vi "Copy_SourceItem.vi"(7 "referencedNonLVTypeMembers in":T1[](array[typedef]), 8 "error in (no error)":errorcluster, 10 "AB_Build.lvclass":refnum<class "AB_Build.lvclass">, 11 "AB_Source_ExportedVI in":refnum<class "AB_Source_ExportedVI.lvclass">) -> (0 "error out":errorcluster, 1 "newFileFlags":T2, 2 "newFileInfo":T3, 3 "AB_Source_ExportedVI out":refnum<class "AB_Source_ExportedVI.lvclass">, 5 "referencedNonLVTypeMembers out":T1[](array[typedef]))   [LabVIEW 2020, in "AB_Source_ExportedVI.lvclass"]
uses:
  <vilib>/AppBuilder/AB_Classes/Source/ExportedVI/AB_Source_ExportedVI.lvclass
  <vilib>/AppBuilder/AB_Classes/Build/AB_Build.lvclass
  <vilib>/AppBuilder/Engine/AB_Engine_New_File_Info.ctl
  <vilib>/AppBuilder/Engine/AB_Engine_New_File_Flags.ctl
  <vilib>/AppBuilder/AB_Source_Referenced_Libray_Files.ctl
  <vilib>/AppBuilder/AB_Classes/Source/VI/AB_Source_VI.lvclass
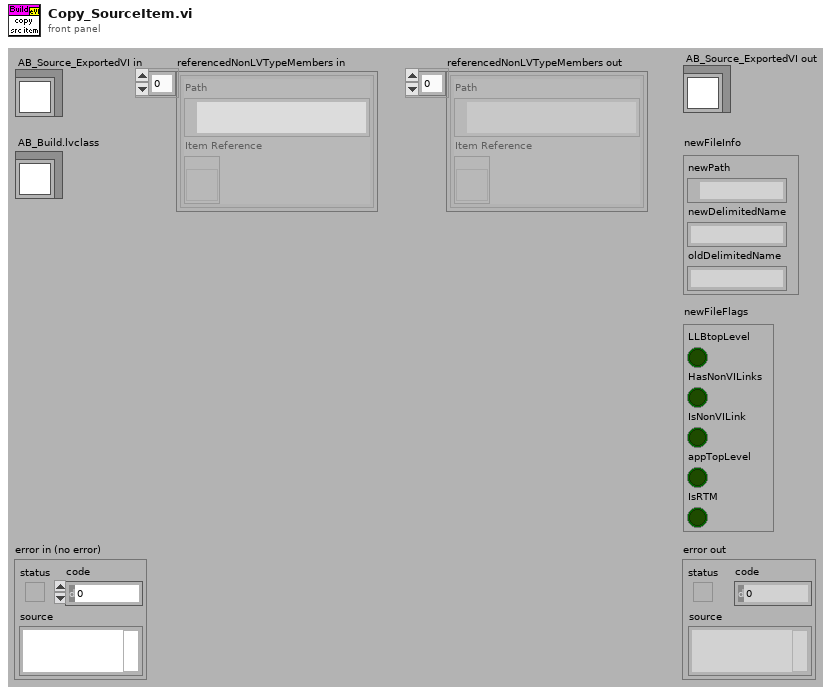
[diagram p1: front panel]
types:
  T1 = typedef "AB_Source_Referenced_Libray_Files.ctl" = cluster{"Path":path, "Item Reference":refnum<vi>}
  T2 = typedef "AB_Engine_New_File_Flags.ctl" = cluster{"LLBtopLevel":bool, "HasNonVILinks":bool, "IsNonVILink":bool, "appTopLevel":bool, "IsRTM":bool}
  T3 = typedef "AB_Engine_New_File_Info.ctl" = cluster{"newPath":path, "newDelimitedName":string, "oldDelimitedName":string}
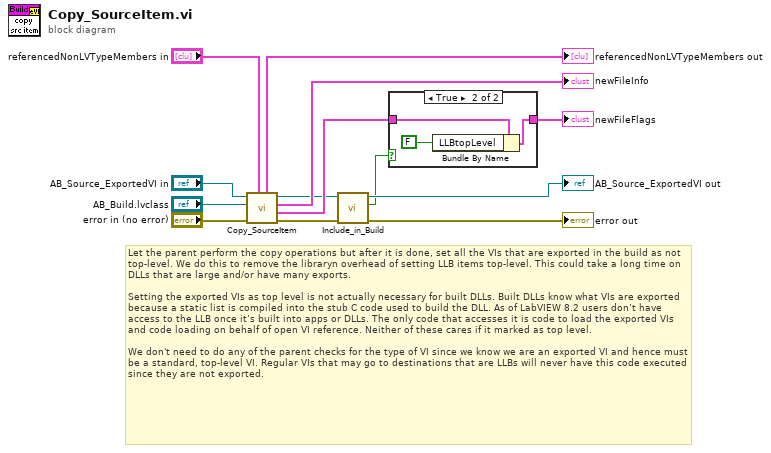
[diagram p0: block diagram]
diagram:
  # "Let the parent perform the copy operations but after it is done, set all the VIs that are exported in the build as not top-level. We do this to remove the libraryn overhead of setting LLB items top-level. This could take a long time on DLLs that are large and/or have many exports.\n\nSetting the exported VIs as top level is not actually necessary for built DLLs. Built DLLs know what VIs are exported because a static list is compiled into the stub C code used to build the DLL. As of LabVIEW 8.2 users don’t have access to the LLB once it’s built into apps or DLLs. The only code that accesses it is code to load the exported VIs and code loading on behalf of open VI reference. Neither of these cares if it marked as top level. \n\nWe don't need to do any of the parent checks for the type of VI since we know we are an exported VI and hence must be a standard, top-level VI. Regular VIs that may go to destinations that are LLBs will never have this code executed since they are not exported."
  n1 = call-parent "Copy_SourceItem.vi"("referencedNonLVTypeMembers in"="referencedNonLVTypeMembers in", "error in (no error)"="error in (no error)", "AB_Build.lvclass"="AB_Build.lvclass", "AB_Source_VI in"="AB_Source_ExportedVI in") -> ("error out"=w5:errorcluster, "newFileFlags"=w7:T2, "newFileInfo"=→"newFileInfo":T3, "AB_Source_VI out"=w3:refnum<class "AB_Source_ExportedVI.lvclass">, "referencedNonLVTypeMembers out"=→"referencedNonLVTypeMembers out":T1[])  [unwired: 3 out]
  n2 = call-dynamic "Include_in_Build.vi"("error in (no error)"=w5, "AB_Source in"=w3) -> ("error out"=→"error out":errorcluster, "includeInBuild"=w1:bool, "AB_Source out"=→"AB_Source_ExportedVI out":refnum<class "AB_Source_ExportedVI.lvclass">)  [unwired: 7 out]
  n3 = case shown="True" w1 {
    tunnel: w7 -> [w14 w17]
    tunnel: [w14 w16] -> w6
    frame False {
    }
    frame True {
      n4 = Bundle By Name(cluster=w17, "LLBtopLevel"=FALSE) -> (w16:T2)
    }
  }
  "newFileFlags" <- w6
